vi "FTW-Test-JSON-Parse.vi"() -> ()   [LabVIEW 2015]
panel:
  out "Passed":bool
  out "Errors":errorcluster[](array[cluster])
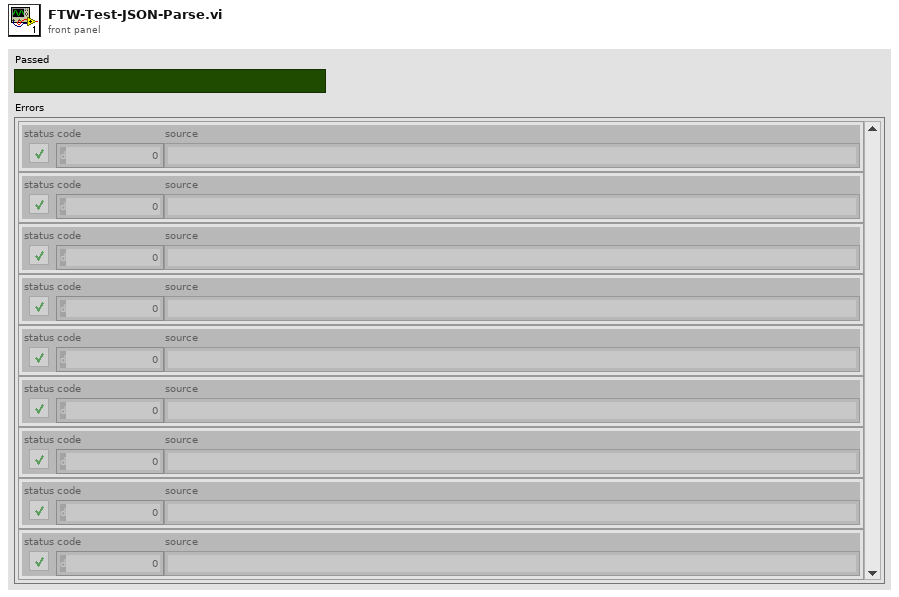
[diagram p1: front panel]
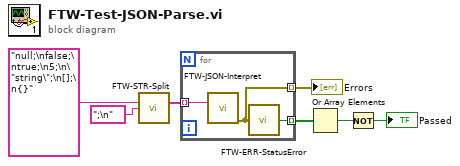
[diagram p0: block diagram]
diagram:
  n1 = call "FTW-STR-Split.vi"("Delimited String"="null;\nfalse;\ntrue;\n5;\n\"string\";\n[];\n{}", "Delimiter"=";\n" ("empty string")) -> ("Array of Strings"=w5:string[])  [unwired: 13 in]
  n2 = for {
    tunnel: w5 -> [w10] mode=indexing
    tunnel: [w9] -> w4 mode=indexing
    tunnel: [w8] -> w3 mode=indexing
    n3 = call "FTW-JSON-Interpret.vi"("JSON String"=w10) -> ("error out"=w9:errorcluster)  [unwired: 12 in, 2 out]
    n4 = call "FTW-ERR-StatusError.vi"("error to check"=w9) -> ("Error?"=w8:bool)
  }
  "Errors" <- w4
  n5 = Or Array Elements(Boolean array=w3) -> (logical OR=w2:bool)
  n6 = Not(x=w2) -> (.not. x?=→"Passed":bool)
